vi "Invalid Name Format.vi"(8 "error in (no error)":errorcluster, 10 "Name":string) -> (0 "error out":errorcluster)   [LabVIEW 2018, in "Application.lvlib" / "Exceptions.lvclass"]
uses:
  Exceptions.lvclass
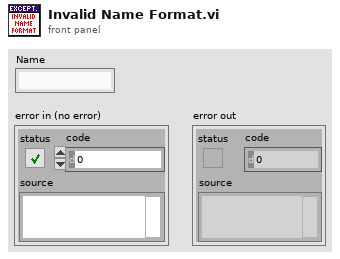
[diagram p1: front panel]
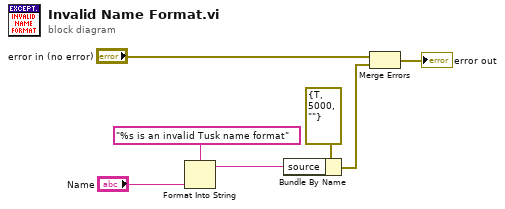
[diagram p0: block diagram]
diagram:
  n1 = Format Into String(format string="%s is an invalid Tusk name format" ("source"), "Name") -> (resulting string=w4:string)  [unwired: 2 in, 1 out]
  n2 = Bundle By Name(cluster=errorcluster {"status"=TRUE, "code"=5000, "source"=""} ("error out"), "source"=w4) -> (w1:errorcluster)
  n3 = Merge Errors("error in (no error)", w1) -> (→"error out":errorcluster)
